vi "z id to string.vi"(8 "error in (no error)":errorcluster, 10 "dst":cluster{}, 11 "zid":cluster{}) -> (0 "error out":errorcluster, 2 "dst out":cluster{})   [LabVIEW 2021, in "zenohc.lvlib"]
doc: "ZENOHC_API void z_id_to_string(const struct z_id_t *zid, struct z_owned_string_t *dst);"
uses:
  zenohc.lvlib
  zenohc.dll
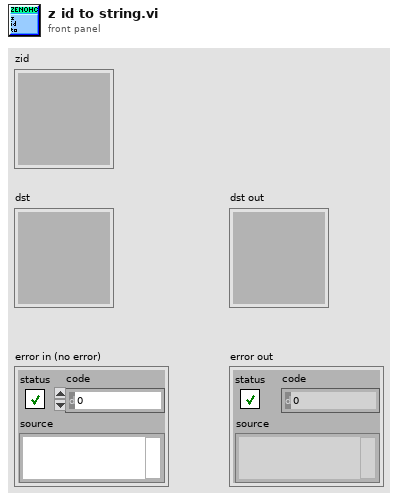
[diagram p1: front panel]
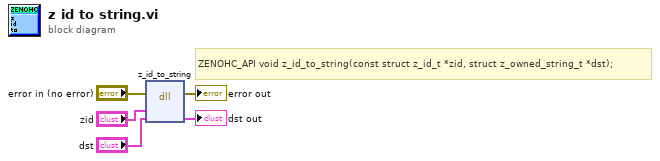
[diagram p0: block diagram]
diagram:
  # "ZENOHC_API void z_id_to_string(const struct z_id_t *zid, struct z_owned_string_t *dst);"
  n1 = dll-call lib="D:/dev/zenoh_labview/zenohc/zenohc.*" fn="z_id_to_string"(error in="error in (no error)", "zid"="zid", "dst"="dst") -> (error out=→"error out":errorcluster, "dst"=→"dst out":cluster{})  [unwired: 4 in, 1 out]
